vi "#65_MAV_MSG_RC_CHANNELS_DECODE.vi"(11 "mavlink_payload":u8[](array[numeric])) -> (3 "RC_CHANNELS":T1)   [LabVIEW 2023]
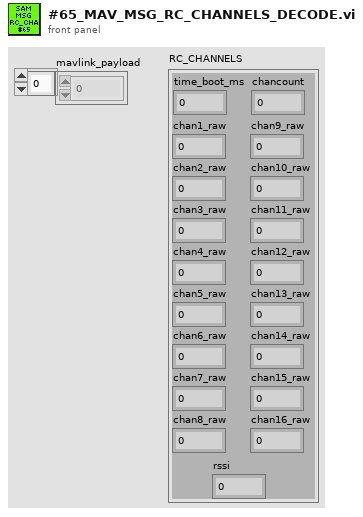
[diagram p1: front panel]
types:
  T1 = cluster{"time_boot_ms":u32, "chancount":u8, "chan1_raw":u16, "chan2_raw":u16, "chan3_raw":u16, "chan4_raw":u16, "chan5_raw":u16, "chan6_raw":u16, "chan7_raw":u16, "chan8_raw":u16, "chan9_raw":u16, "chan10_raw":u16, "chan11_raw":u16, "chan12_raw":u16, "chan13_raw":u16, "chan14_raw":u16, "chan15_raw":u16, "chan16_raw":u16, "rssi":u8}
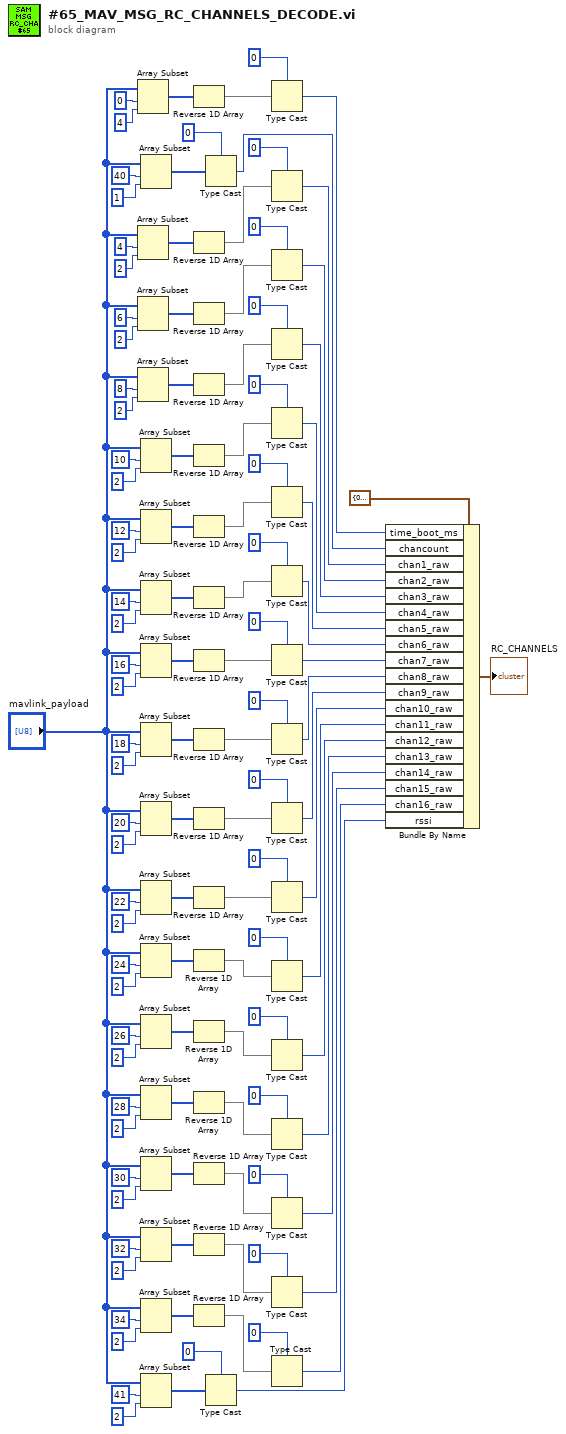
[diagram p0: block diagram]
diagram:
  n1 = Array Subset(array="mavlink_payload", index=0 ("Index"), length=4) -> (w114:u8[])
  n2 = Array Subset(array="mavlink_payload", index=4 ("Index"), length=2) -> (w102:u8[])
  n3 = Array Subset(array="mavlink_payload", index=6 ("Index"), length=2) -> (w96:u8[])
  n4 = Array Subset(array="mavlink_payload", index=8 ("Index"), length=2) -> (w90:u8[])
  n5 = Array Subset(array="mavlink_payload", index=40 ("Index"), length=1) -> (w1:u8[])
  n6 = Array Subset(array="mavlink_payload", index=10 ("Index"), length=2) -> (w84:u8[])
  n7 = Array Subset(array="mavlink_payload", index=12 ("Index"), length=2) -> (w78:u8[])
  n8 = Array Subset(array="mavlink_payload", index=14 ("Index"), length=2) -> (w72:u8[])
  n9 = Array Subset(array="mavlink_payload", index=16 ("Index"), length=2) -> (w66:u8[])
  n10 = Array Subset(array="mavlink_payload", index=18 ("Index"), length=2) -> (w60:u8[])
  n11 = Array Subset(array="mavlink_payload", index=20 ("Index"), length=2) -> (w54:u8[])
  n12 = Array Subset(array="mavlink_payload", index=22 ("Index"), length=2) -> (w48:u8[])
  n13 = Array Subset(array="mavlink_payload", index=24 ("Index"), length=2) -> (w42:u8[])
  n14 = Array Subset(array="mavlink_payload", index=26 ("Index"), length=2) -> (w36:u8[])
  n15 = Array Subset(array="mavlink_payload", index=28 ("Index"), length=2) -> (w30:u8[])
  n16 = Array Subset(array="mavlink_payload", index=30 ("Index"), length=2) -> (w24:u8[])
  n17 = Array Subset(array="mavlink_payload", index=32 ("Index"), length=2) -> (w18:u8[])
  n18 = Array Subset(array="mavlink_payload", index=34 ("Index"), length=2) -> (w12:u8[])
  n19 = Array Subset(array="mavlink_payload", index=41 ("Index"), length=2) -> (w3:u8[])
  n20 = Reverse 1D Array(array=w114) -> (reversed array=w113:u8[])
  n21 = Reverse 1D Array(array=w102) -> (reversed array=w101:u8[])
  n22 = Reverse 1D Array(array=w96) -> (reversed array=w95:u8[])
  n23 = Reverse 1D Array(array=w90) -> (reversed array=w89:u8[])
  n24 = Reverse 1D Array(array=w84) -> (reversed array=w83:u8[])
  n25 = Reverse 1D Array(array=w78) -> (reversed array=w77:u8[])
  n26 = Reverse 1D Array(array=w72) -> (reversed array=w71:u8[])
  n27 = Reverse 1D Array(array=w66) -> (reversed array=w65:u8[])
  n28 = Reverse 1D Array(array=w60) -> (reversed array=w59:u8[])
  n29 = Reverse 1D Array(array=w54) -> (reversed array=w53:u8[])
  n30 = Reverse 1D Array(array=w48) -> (reversed array=w47:u8[])
  n31 = Reverse 1D Array(array=w42) -> (reversed array=w41:u8[])
  n32 = Reverse 1D Array(array=w36) -> (reversed array=w35:u8[])
  n33 = Reverse 1D Array(array=w30) -> (reversed array=w29:u8[])
  n34 = Reverse 1D Array(array=w24) -> (reversed array=w23:u8[])
  n35 = Reverse 1D Array(array=w18) -> (reversed array=w17:u8[])
  n36 = Reverse 1D Array(array=w12) -> (reversed array=w11:u8[])
  n37 = Type Cast(type=u8 0 ("Index"), x=w1) -> (*(type *) &x=w104:u8)
  n38 = Type Cast(type=u8 0 ("Index"), x=w3) -> (*(type *) &x=w2:u8)
  n39 = Type Cast(type=u32 0 ("Index"), x=w113) -> (*(type *) &x=w108:u32)
  n40 = Type Cast(type=u16 0 ("Index"), x=w101) -> (*(type *) &x=w98:u16)
  n41 = Type Cast(type=u16 0 ("Index"), x=w95) -> (*(type *) &x=w92:u16)
  n42 = Type Cast(type=u16 0 ("Index"), x=w89) -> (*(type *) &x=w86:u16)
  n43 = Type Cast(type=u16 0 ("Index"), x=w83) -> (*(type *) &x=w80:u16)
  n44 = Type Cast(type=u16 0 ("Index"), x=w77) -> (*(type *) &x=w74:u16)
  n45 = Type Cast(type=u16 0 ("Index"), x=w71) -> (*(type *) &x=w68:u16)
  n46 = Type Cast(type=u16 0 ("Index"), x=w65) -> (*(type *) &x=w62:u16)
  n47 = Type Cast(type=u16 0 ("Index"), x=w59) -> (*(type *) &x=w56:u16)
  n48 = Type Cast(type=u16 0 ("Index"), x=w53) -> (*(type *) &x=w50:u16)
  n49 = Type Cast(type=u16 0 ("Index"), x=w47) -> (*(type *) &x=w44:u16)
  n50 = Type Cast(type=u16 0 ("Index"), x=w41) -> (*(type *) &x=w38:u16)
  n51 = Type Cast(type=u16 0 ("Index"), x=w35) -> (*(type *) &x=w32:u16)
  n52 = Type Cast(type=u16 0 ("Index"), x=w29) -> (*(type *) &x=w26:u16)
  n53 = Type Cast(type=u16 0 ("Index"), x=w23) -> (*(type *) &x=w20:u16)
  n54 = Type Cast(type=u16 0 ("Index"), x=w17) -> (*(type *) &x=w14:u16)
  n55 = Type Cast(type=u16 0 ("Index"), x=w11) -> (*(type *) &x=w8:u16)
  n56 = Bundle By Name(cluster=T1 {"time_boot_ms"=0, "chancount"=0, "chan1_raw"=0, "chan2_raw"=0, "chan3_raw"=0, "chan4_raw"=0, "chan5_raw"=0, "chan6_raw"=0, "chan7_raw"=0, "chan8_raw"=0, "chan9_raw"=0, "chan10_raw"=0, "chan11_raw"=0, "chan12_raw"=0, "chan13_raw"=0, "chan14_raw"=0, "chan15_raw"=0, "chan16_raw"=0, "rssi"=0} ("RC_CHANNELS"), "time_boot_ms"=w108, "chancount"=w104, "chan1_raw"=w98, "chan2_raw"=w92, "chan3_raw"=w86, "chan4_raw"=w80, "chan5_raw"=w74, "chan6_raw"=w68, "chan7_raw"=w62, "chan8_raw"=w56, "chan9_raw"=w50, "chan10_raw"=w44, "chan11_raw"=w38, "chan12_raw"=w32, "chan13_raw"=w26, "chan14_raw"=w20, "chan15_raw"=w14, "chan16_raw"=w8, "rssi"=w2) -> (→"RC_CHANNELS":T1)
